vi "save_config_file.vi"(8 "error in (no error)":errorcluster, 11 "GenericPlugin in":refnum<class "DataCollectionDL090215.lvclass">) -> (0 "error out":errorcluster, 3 "GenericPlugin out":refnum<class "DataCollectionDL090215.lvclass">)   [LabVIEW 2010, in "DataCollectionDL090215.lvclass"]
uses:
  DataCollectionDL090215.lvclass
  DataCollectionDL090215.lvclass/DataCollectionDL090215.ctl
  DataCollectionDL091104Scaffold/DataCollectionDL091104Scaffold/DataCollectionDL091104Scaffold.lvclass
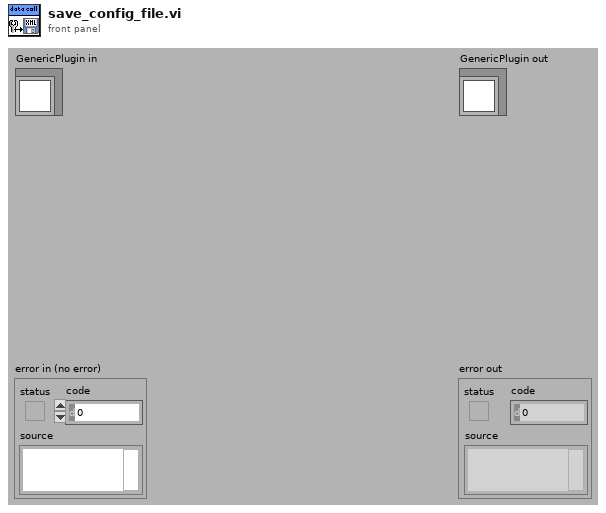
[diagram p1: front panel]
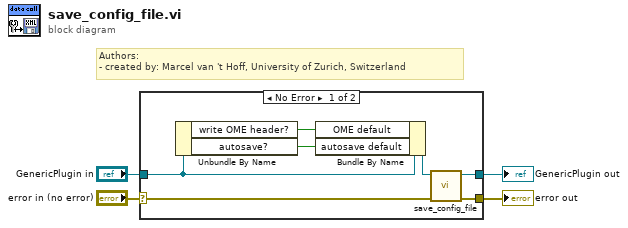
[diagram p0: block diagram]
diagram:
  # "Authors: \n- created by: Marcel van 't Hoff, University of Zurich, Switzerland"
  n1 = case shown="No Error" "error in (no error)" {
    selector: "error in (no error)" -> [w9 w12]
    tunnel: [w11 w12] -> w4
    tunnel: [w10 w13] -> w3
    tunnel: "GenericPlugin in" -> [w8 w13]
    frame No Error {
      n2 = Unbundle By Name(w8) -> ("write OME header?"=w6:bool, "autosave?"=w5:bool)
      n3 = Bundle By Name(cluster=w8, "OME default"=w6, "autosave default"=w5) -> (w7:refnum<class "DataCollectionDL090215.lvclass">)
      n4 = call-parent "save_config_file.vi"("error in (no error)"=w9, "GenericPlugin in"=w7) -> ("error out"=w11:errorcluster, "GenericPlugin out"=w10:refnum<class "DataCollectionDL090215.lvclass">)  [unwired: 8 in]
    }
    frame Error {
    }
  }
  "error out" <- w4
  "GenericPlugin out" <- w3
